vi "SetOutput.vi"(8 "error in (no error)":errorcluster, 9 "Boolean":bool=TRUE, 10 "Index":i32, 11 "DMC1000B in":refnum<class "DMC1000B.lvclass">) -> (0 "error out":errorcluster, 1 "life+1":bool, 3 "DMC1000B out":refnum<class "DMC1000B.lvclass">)   [LabVIEW 2019, in "DMC1000B.lvclass"]
uses:
  DMC1000B.lvclass
  LLB/DMC1000B/Dmc1000/Dmc1000.lvlib
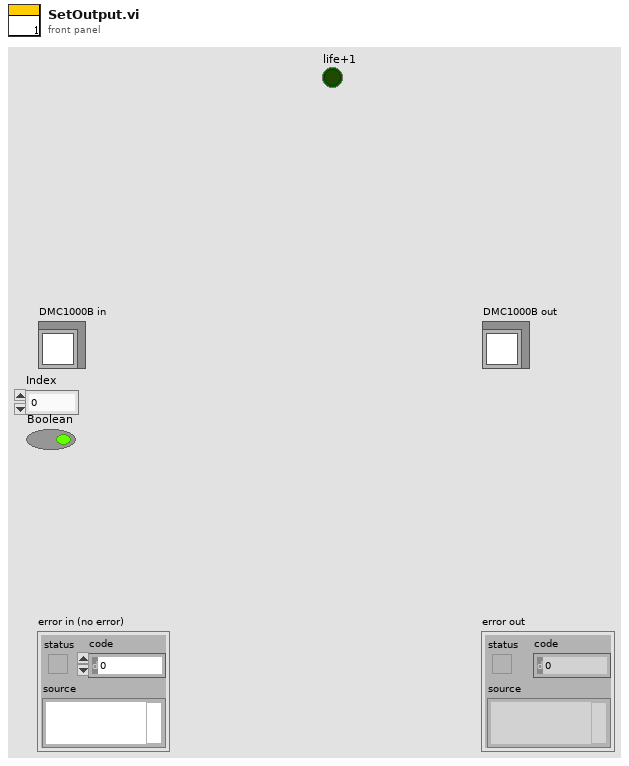
[diagram p1: front panel]
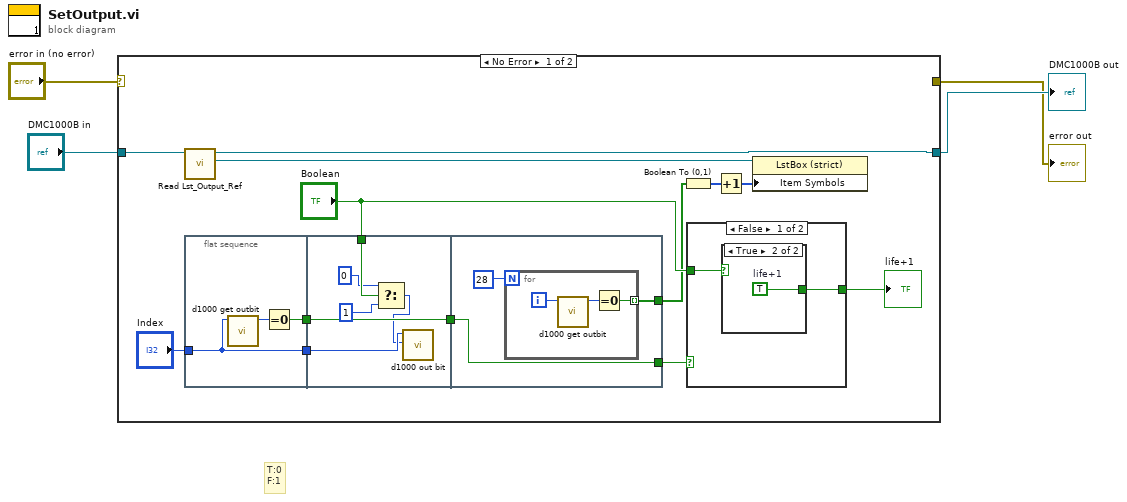
[diagram p0: block diagram]
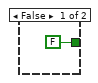
[diagram p2: hidden frame]
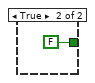
[diagram p3: hidden frame]
diagram:
  # "T:0\nF:1"
  n1 = case shown="No Error" "error in (no error)" {
    selector: "error in (no error)" -> [_ w39]
    tunnel: "DMC1000B in" -> [w10 w38]
    tunnel: [_ w39] -> w1
    tunnel: [w5 w38] -> w2
    frame No Error {
      n2 = call-dynamic "Read Lst_Output_Ref.vi"("IOCard in"=w10) -> ("Lst_Output_Ref"=w9:refnum<vi>, "IOCard out"=w5:refnum<class "DMC1000B.lvclass">)  [unwired: 8 in, 1 out]
      n3 = flat-sequence {
        tunnel: "Index" -> [w18]
        tunnel: [w20] -> w15
        tunnel: [w18] -> w12
        tunnel: w15 -> [w26]
        tunnel: "Boolean" -> [w24]
        tunnel: w12 -> [w25]
        tunnel: [w26] -> w11
        tunnel: [w29] -> w16
        tunnel: w11 -> [w29]
        tunnel: [w27] -> w8
        frame #0 {
          n4 = call "d1000 get outbit.vi"("BitNo"=w18) -> ("function return"=w19:u32)  [unwired: 10 in]
          n5 = Equal To 0?(x=w19) -> (x = 0?=w20:bool)
        }
        frame #1 {
          n6 = Select(t=0, s=w24, f=1) -> (s? t:f=w21:i32)
          n7 = call "d1000 out bit.vi"("BitData"=w21, "BitNo"=w25) -> ()  [unwired: 9 in, 1 out]
        }
        frame #2 {
          n8 = for {
            N: 28 -> [_]
            tunnel: [w30] -> w27 mode=indexing
            i -> [w31]
            n9 = call "d1000 get outbit.vi"("BitNo"=w31) -> ("function return"=w32:u32)  [unwired: 10 in]
            n10 = Equal To 0?(x=w32) -> (x = 0?=w30:bool)
          }
        }
      }
      n11 = Boolean To (0,1)(Boolean=w8) -> (0, 1=w7:i16[])
      n12 = case shown="False" w16 {
        tunnel: "Boolean" -> [w34 _]
        tunnel: [w33 FALSE ("life+1")] -> w17
        frame False {
          n13 = case shown="True" w34 {
            tunnel: [FALSE ("life+1") w36] -> w33
            frame False {
            }
            frame True {
              w36 = TRUE  # life+1
            }
          }
        }
        frame True {
        }
      }
      "life+1" <- w17
      n14 = Increment(x=w7) -> (x+1=w6:i16[])
      n15 = property class="LstBox (strict)"(reference=w9, "Item Symbols"=w6) -> ()  [unwired: 1 in, 2 out]
    }
    frame Error {
    }
  }
  "error out" <- w1
  "DMC1000B out" <- w2
